vi "REPEORT.CAMBIO LINEA.vi"(2 "Text Out":string) -> (7 "String":string)   [LabVIEW 2019]
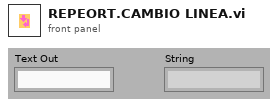
[diagram p1: front panel]
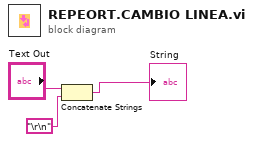
[diagram p0: block diagram]
diagram:
  n1 = Concatenate Strings("Text Out", "\r\n") -> (→"String":string)
